vi "Config_PXDAC4800.vi"(0 "NumBoard":u32=1, 5 "Config":T1={"Clock source"=enum."1200 MHz", "Active channel"=enum."Single channel - Ch1", "Trigger direction"=enum."Positive (Rising edge)", "Trigger mode"=enum."Per trigger", "External Trigger enable"=FALSE, "Dac sample size"=enum."14 Bits LSB\n", "Dac sample format"=enum."Unsigned", "ClkDiv1"=1, "ClkDiv2"=1, "Output voltage level - Ch1"=1023, "Output voltage level - Ch2"=1023, "Output voltage level - Ch3"=1023, "Output voltage level - Ch4"=1023} {"Output voltage level - Ch4" min=1 max=1023 step=1 scale=0.0..1023.0; "Output voltage level - Ch3" min=1 max=1023 step=1 scale=0.0..1023.0; "Output voltage level - Ch2" min=1 max=1023 step=1 scale=0.0..1023.0; "Output voltage level - Ch1" min=1 max=1023 step=1 scale=0.0..1023.0}) -> (6 "Handle":u32, 8 "Serial num":u32, 10 "Status":i32, 15 "Error/output message":string)   [LabVIEW 2016]
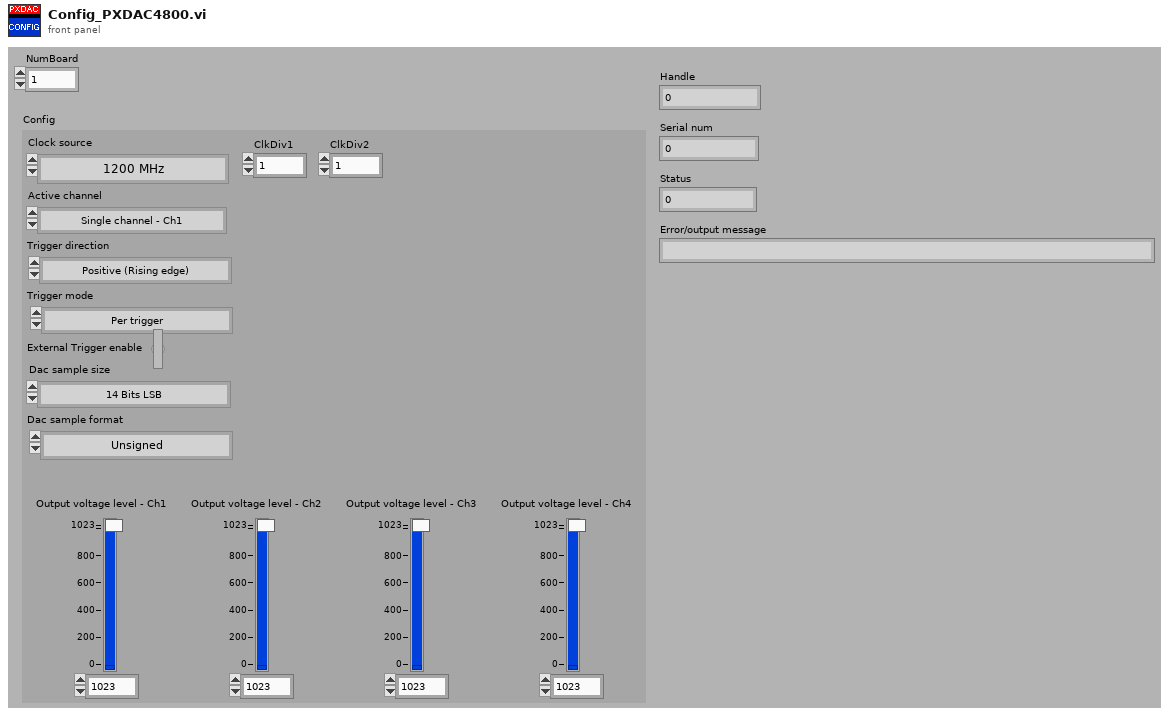
[diagram p1: front panel]
types:
  T1 = cluster{"Clock source":enum16{"1200 MHz", "900 MHz", "External"}, "Active channel":enum16{"Four channel", "Dual channel - Ch1 & Ch2", "Dual channel - Ch3 & Ch4", "Single channel - Ch1", "Single channel - Ch2", "Single channel - Ch3", "Single channel - Ch4"}, "Trigger direction":enum16{"Positive (Rising edge)", "Negative (Falling edge)"}, "Trigger mode":enum16{"Per trigger", "Continuous", "Single shot"}, "External Trigger enable":bool, "Dac sample size":enum16{"8 bits", "14 bits MSB", "14 Bits LSB\n"}, "Dac sample format":enum16{"Unsigned", "Signed"}, "ClkDiv1":u32, "ClkDiv2":u32, "Output voltage level - Ch1":u32, "Output voltage level - Ch2":u32, "Output voltage level - Ch3":u32, "Output voltage level - Ch4":u32}
  T2 = enum16{"Connect", "GetSerialNumber", "SetActiveChannelMaskXD48", "SetPlaybackClockSourceXD48", "SetClockDivider1XD48", "SetClockDivider2XD48", "SetOutputVoltageCh1XD48", "SetOutputVoltageCh2XD48", "SetOutputVoltageCh3XD48", "SetOutputVoltageCh4XD48", "SetDacSampleFormatXD48", "SetDacSampleSizeXD48", "SetExternalTriggerEnableXD48", "SetExternalTriggerDirXD48", "SetTriggerModeXD48", "Disconnect"}
  T3 = enum16{"Four channel", "Dual channel - Ch1 & Ch2", "Dual channel - Ch3 & Ch4", "Single channel - Ch1", "Single channel - Ch2", "Single channel - Ch3", "Single channel - Ch4"}
  T4 = enum16{"Positive (Rising edge)", "Negative (Falling edge)"}
  T5 = enum16{"Per trigger", "Continuous", "Single shot"}
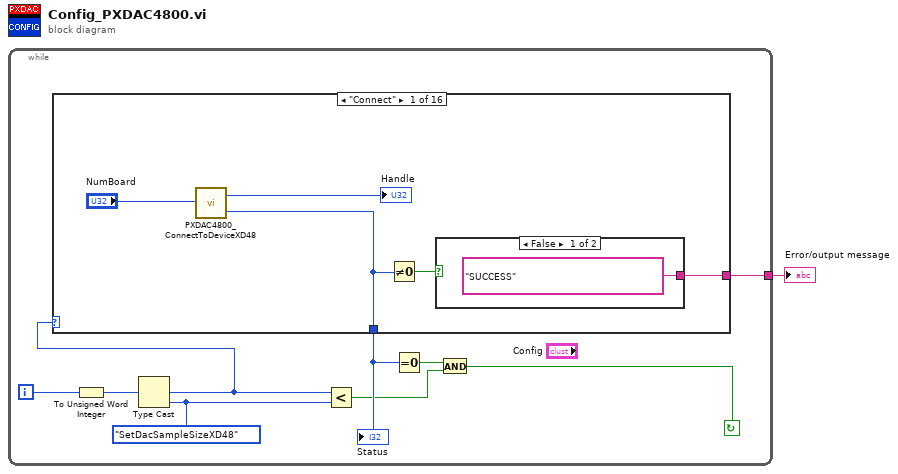
[diagram p0: block diagram]
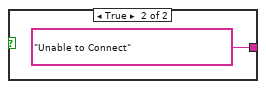
[diagram p2: hidden frame]
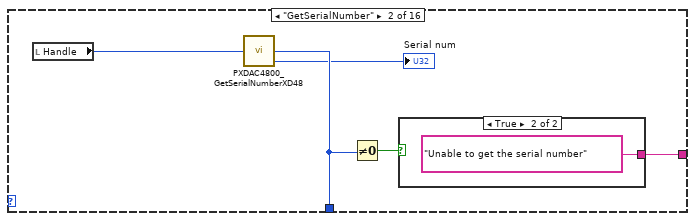
[diagram p3: hidden frame]
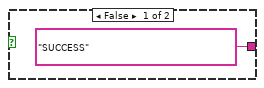
[diagram p4: hidden frame]
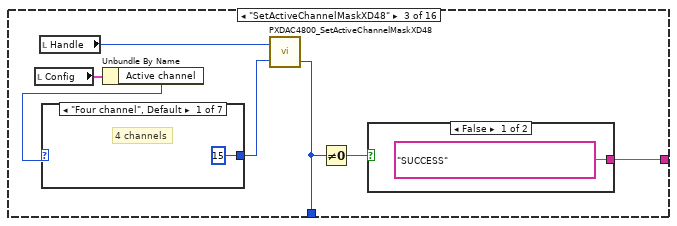
[diagram p5: hidden frame]
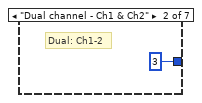
[diagram p6: hidden frame]
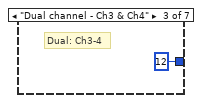
[diagram p7: hidden frame]
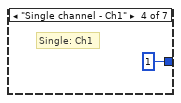
[diagram p8: hidden frame]
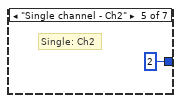
[diagram p9: hidden frame]
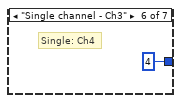
[diagram p10: hidden frame]
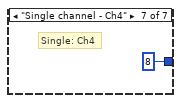
[diagram p11: hidden frame]
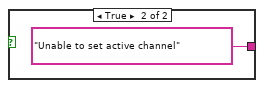
[diagram p12: hidden frame]
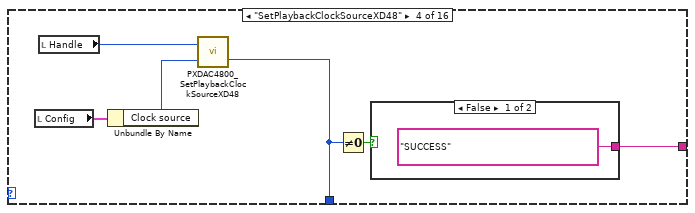
[diagram p13: hidden frame]
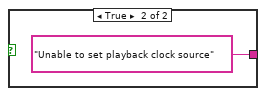
[diagram p14: hidden frame]
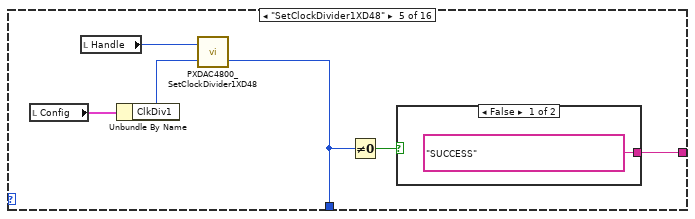
[diagram p15: hidden frame]
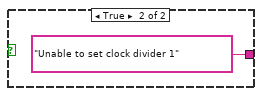
[diagram p16: hidden frame]
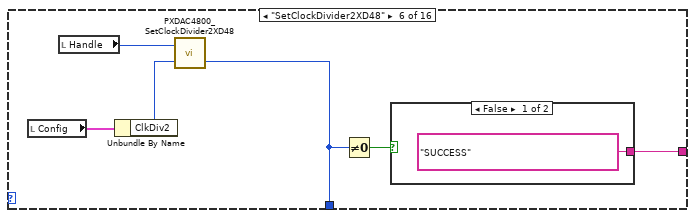
[diagram p17: hidden frame]
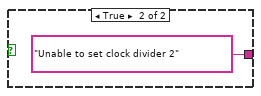
[diagram p18: hidden frame]
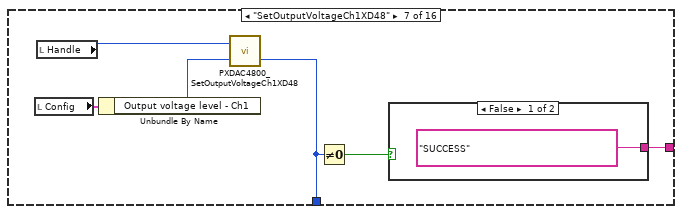
[diagram p19: hidden frame]
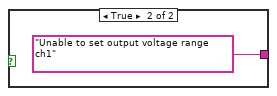
[diagram p20: hidden frame]
diagram:
  n1 = while {
    tunnel: [w2] -> w1
    i -> [w10]
    stop <- w3 continue-if-true
    w7 = T2."SetDacSampleSizeXD48"
    n2 = To Unsigned Word Integer(number=w10) -> (unsigned 16bit integer=w9:u16)
    n3 = Type Cast(type=w7, x=w9) -> (*(type *) &x=w8:T2)
    n4 = case shown="\"Connect\"" w8 {
      tunnel: [w11 w20 w29 w44 w51 w59 w67 w75 w83 w91 w99 w107 w115 w126 w134 w140] -> w6
      tunnel: [w14 w21 w30 w45 w53 w61 w69 w77 w85 w93 w101 w109 w118 w128 w136 w143] -> w2
      frame "Connect" {
        n5 = call "PXDAC4800_ConnectToDeviceXD48.vi"("brdNum"="NumBoard") -> ("Handle Out"=→"Handle":i32, "Status"=w11:i32)
        n6 = Not Equal To 0?(x=w11) -> (x != 0?=w15:bool)
        n7 = case shown="False" w15 {
          tunnel: ["SUCCESS" "Unable to Connect"] -> w14
          frame False {
          }
          frame True {
          }
        }
      }
      frame "GetSerialNumber" {
        (unwired) "Unable to get serial"
        n8 = local read "Handle"() -> (w18:u32)
        n9 = call "PXDAC4800_GetSerialNumberXD48.vi"("Handle"=w18) -> ("Status"=w20:i32, "Serial num"=→"Serial num":i32)  [unwired: 1 out]
        n10 = Not Equal To 0?(x=w20) -> (x != 0?=w22:bool)
        n11 = case shown="True" w22 {
          tunnel: ["SUCCESS" "Unable to get the serial number"] -> w21
          frame False {
          }
          frame True {
          }
        }
      }
      frame "SetActiveChannelMaskXD48" {
        n12 = local read "Config"() -> (w26:T1)
        n13 = local read "Handle"() -> (w28:u32)
        n14 = Unbundle By Name(w26) -> ("Active channel"=w25:T3)
        n15 = case shown="\"Four channel\", Default" w25 {
          tunnel: [15 3 12 1 2 4 8] -> w27
          frame "Four channel", Default {
            # "4 channels"
          }
          frame "Dual channel - Ch1 & Ch2" {
            # "Dual: Ch1-2"
          }
          frame "Dual channel - Ch3 & Ch4" {
            # "Dual: Ch3-4"
          }
          frame "Single channel - Ch1" {
            # "Single: Ch1"
          }
          frame "Single channel - Ch2" {
            # "Single: Ch2"
          }
          frame "Single channel - Ch3" {
            # "Single: Ch4"
          }
          frame "Single channel - Ch4" {
            # "Single: Ch4"
          }
        }
        n16 = call "PXDAC4800_SetActiveChannelMaskXD48.vi"("Value"=w27, "Handle"=w28) -> ("Status"=w29:i32)  [unwired: 1 out]
        n17 = Not Equal To 0?(x=w29) -> (x != 0?=w31:bool)
        n18 = case shown="False" w31 {
          tunnel: ["SUCCESS" "Unable to set active channel"] -> w30
          frame False {
          }
          frame True {
          }
        }
      }
      frame "SetPlaybackClockSourceXD48" {
        n19 = local read "Config"() -> (w42:T1)
        n20 = local read "Handle"() -> (w43:u32)
        n21 = Unbundle By Name(w42) -> ("Clock source"=w41:enum16{"1200 MHz", "900 MHz", "External"})
        n22 = call "PXDAC4800_SetPlaybackClockSourceXD48.vi"("Value"=w41, "Handle"=w43) -> ("Status"=w44:i32)  [unwired: 1 out]
        n23 = Not Equal To 0?(x=w44) -> (x != 0?=w46:bool)
        n24 = case shown="False" w46 {
          tunnel: ["SUCCESS" "Unable to set playback clock source"] -> w45
          frame False {
          }
          frame True {
          }
        }
      }
      frame "SetClockDivider1XD48" {
        n25 = local read "Config"() -> (w50:T1)
        n26 = local read "Handle"() -> (w52:u32)
        n27 = Unbundle By Name(w50) -> ("ClkDiv1"=w49:u32)
        n28 = call "PXDAC4800_SetClockDivider1XD48.vi"("Div"=w49, "Handle"=w52) -> ("Status"=w51:i32)  [unwired: 1 out]
        n29 = Not Equal To 0?(x=w51) -> (x != 0?=w54:bool)
        n30 = case shown="False" w54 {
          tunnel: ["SUCCESS" "Unable to set clock divider 1"] -> w53
          frame False {
          }
          frame True {
          }
        }
      }
      frame "SetClockDivider2XD48" {
        n31 = local read "Config"() -> (w58:T1)
        n32 = local read "Handle"() -> (w60:u32)
        n33 = Unbundle By Name(w58) -> ("ClkDiv2"=w57:u32)
        n34 = call "PXDAC4800_SetClockDivider2XD48.vi"("Div"=w57, "Handle"=w60) -> ("Status"=w59:i32)  [unwired: 1 out]
        n35 = Not Equal To 0?(x=w59) -> (x != 0?=w62:bool)
        n36 = case shown="False" w62 {
          tunnel: ["SUCCESS" "Unable to set clock divider 2"] -> w61
          frame False {
          }
          frame True {
          }
        }
      }
      frame "SetOutputVoltageCh1XD48" {
        n37 = local read "Config"() -> (w66:T1)
        n38 = local read "Handle"() -> (w68:u32)
        n39 = Unbundle By Name(w66) -> ("Output voltage level - Ch1"=w65:u32)
        n40 = call "PXDAC4800_SetOutputVoltageCh1XD48.vi"("Value"=w65, "Handle"=w68) -> ("Status"=w67:i32)  [unwired: 1 out]
        n41 = Not Equal To 0?(x=w67) -> (x != 0?=w70:bool)
        n42 = case shown="False" w70 {
          tunnel: ["SUCCESS" "Unable to set output voltage range ch1"] -> w69
          frame False {
          }
          frame True {
          }
        }
      }
      frame "SetOutputVoltageCh2XD48" {
        n43 = local read "Config"() -> (w74:T1)
        n44 = local read "Handle"() -> (w76:u32)
        n45 = Unbundle By Name(w74) -> ("Output voltage level - Ch2"=w73:u32)
        n46 = call "PXDAC4800_SetOutputVoltageCh2XD48.vi"("Value"=w73, "Handle"=w76) -> ("Status"=w75:i32)  [unwired: 1 out]
        n47 = Not Equal To 0?(x=w75) -> (x != 0?=w78:bool)
        n48 = case shown="False" w78 {
          tunnel: ["SUCCESS" "Unable to set output voltage range ch2"] -> w77
          frame False {
          }
          frame True {
          }
        }
      }
      frame "SetOutputVoltageCh3XD48" {
        n49 = local read "Config"() -> (w82:T1)
        n50 = local read "Handle"() -> (w84:u32)
        n51 = Unbundle By Name(w82) -> ("Output voltage level - Ch3"=w81:u32)
        n52 = call "PXDAC4800_SetOutputVoltageCh3XD48.vi"("Value"=w81, "Handle"=w84) -> ("Status"=w83:i32)  [unwired: 1 out]
        n53 = Not Equal To 0?(x=w83) -> (x != 0?=w86:bool)
        n54 = case shown="False" w86 {
          tunnel: ["SUCCESS" "Unable to set output voltage range ch3"] -> w85
          frame False {
          }
          frame True {
          }
        }
      }
      frame "SetOutputVoltageCh4XD48" {
        n55 = local read "Config"() -> (w90:T1)
        n56 = local read "Handle"() -> (w92:u32)
        n57 = Unbundle By Name(w90) -> ("Output voltage level - Ch4"=w89:u32)
        n58 = call "PXDAC4800_SetOutputVoltageCh4XD48.vi"("Value"=w89, "Handle"=w92) -> ("Status"=w91:i32)  [unwired: 1 out]
        n59 = Not Equal To 0?(x=w91) -> (x != 0?=w94:bool)
        n60 = case shown="False" w94 {
          tunnel: ["SUCCESS" "Unable to set output voltage range ch4"] -> w93
          frame False {
          }
          frame True {
          }
        }
      }
      frame "SetDacSampleFormatXD48" {
        n61 = local read "Config"() -> (w98:T1)
        n62 = local read "Handle"() -> (w100:u32)
        n63 = Unbundle By Name(w98) -> ("Dac sample format"=w97:enum16{"Unsigned", "Signed"})
        n64 = call "PXDAC4800_SetDacSampleFormatXD48.vi"("Value"=w97, "Handle"=w100) -> ("Status"=w99:i32)  [unwired: 1 out]
        n65 = Not Equal To 0?(x=w99) -> (x != 0?=w102:bool)
        n66 = case shown="False" w102 {
          tunnel: ["SUCCESS" "Unable to set Dac sample format"] -> w101
          frame False {
          }
          frame True {
          }
        }
      }
      frame "SetDacSampleSizeXD48" {
        n67 = local read "Config"() -> (w106:T1)
        n68 = local read "Handle"() -> (w108:u32)
        n69 = Unbundle By Name(w106) -> ("Dac sample size"=w105:enum16{"8 bits", "14 bits MSB", "14 Bits LSB\n"})
        n70 = call "PXDAC4800_SetDacSampleSizeXD48.vi"("Value"=w105, "Handle"=w108) -> ("Status"=w107:i32)  [unwired: 1 out]
        n71 = Not Equal To 0?(x=w107) -> (x != 0?=w110:bool)
        n72 = case shown="False" w110 {
          tunnel: ["SUCCESS" "Unable to set sample size"] -> w109
          frame False {
          }
          frame True {
          }
        }
      }
      frame "SetExternalTriggerEnableXD48" {
        n73 = local read "Config"() -> (w114:T1)
        n74 = local read "Handle"() -> (w117:u32)
        n75 = Unbundle By Name(w114) -> ("External Trigger enable"=w113:bool)
        n76 = case shown="False" w113 {
          tunnel: [0 1] -> w116
          frame False {
          }
          frame True {
          }
        }
        n77 = call "PXDAC4800_SetExternalTriggerEnableXD48.vi"("bEnable"=w116, "Handle"=w117) -> ("Status"=w115:i32)  [unwired: 1 out]
        n78 = Not Equal To 0?(x=w115) -> (x != 0?=w119:bool)
        n79 = case shown="False" w119 {
          tunnel: ["SUCCESS" "Unable to set external trigger enable"] -> w118
          frame False {
          }
          frame True {
          }
        }
      }
      frame "SetExternalTriggerDirXD48" {
        n80 = local read "Config"() -> (w125:T1)
        n81 = local read "Handle"() -> (w127:u32)
        n82 = Unbundle By Name(w125) -> ("Trigger direction"=w124:T4)
        n83 = call "PXDAC4800_SetExternalTriggerDirXD48.vi"("Value"=w124, "Handle"=w127) -> ("Status"=w126:i32)  [unwired: 1 out]
        n84 = Not Equal To 0?(x=w126) -> (x != 0?=w129:bool)
        n85 = case shown="False" w129 {
          tunnel: ["SUCCESS" "Unable to set external trigger direction"] -> w128
          frame False {
          }
          frame True {
          }
        }
      }
      frame "SetTriggerModeXD48" {
        n86 = local read "Config"() -> (w133:T1)
        n87 = local read "Handle"() -> (w135:u32)
        n88 = Unbundle By Name(w133) -> ("Trigger mode"=w132:T5)
        n89 = call "PXDAC4800_SetTriggerModeXD48.vi"("Value"=w132, "Handle"=w135) -> ("Status"=w134:i32)  [unwired: 1 out]
        n90 = Not Equal To 0?(x=w134) -> (x != 0?=w137:bool)
        n91 = case shown="False" w137 {
          tunnel: ["SUCCESS" "Unable to set trigger mode"] -> w136
          frame False {
          }
          frame True {
          }
        }
      }
      frame "Disconnect" {
        n92 = local read "Handle"() -> (w141:u32)
        n93 = call "PXDAC4800_DisconnectToDeviceXD48.vi"("Handle"=w141) -> ("Status"=w140:i32)
        n94 = Not Equal To 0?(x=w140) -> (x != 0?=w142:bool)
        n95 = case shown="False" w142 {
          tunnel: ["SUCCESS" "Unable to disconnect"] -> w143
          frame False {
          }
          frame True {
          }
        }
      }
    }
    "Status" <- w6
    n96 = Less?(x=w8, y=w7) -> (x < y?=w4:bool)
    n97 = Equal To 0?(x=w6) -> (x = 0?=w5:bool)
    n98 = And(x=w5, y=w4) -> (x .and. y?=w3:bool)
  }
  "Error/output message" <- w1
